vi "place_cheese_in_maze.vi"(1 "Array in":T1[][](array[typedef])) -> (0 "Array out":T1[][](array[typedef]))   [LabVIEW 2016]
doc: "Searches for the last open row of last column in the maze the places the cheese in.\n\nMuhannad Alghamdi\nCSUSB Physics 350"
uses:
  typedefs/cell_typedef.ctl
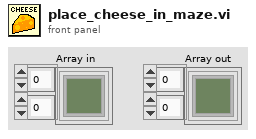
[diagram p1: front panel]
types:
  T1 = typedef "cell_typedef.ctl" = cluster{"open":bool, "runner":u16}
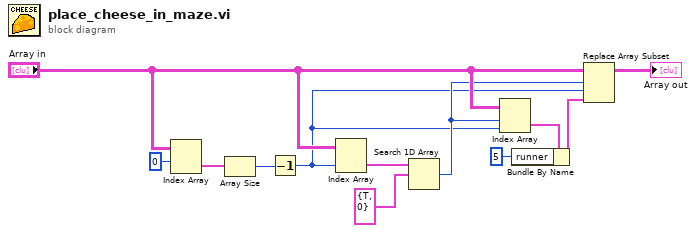
[diagram p0: block diagram]
diagram:
  n1 = Index Array(array="Array in", index (row)=0) -> (element=w6:T1[])  [unwired: 1 in]
  n2 = Array Size(array=w6) -> (size(s)=w7:i32)
  n3 = Decrement(x=w7) -> (x-1=w9:i32)
  n4 = Index Array(array="Array in", index (col)=w9) -> (element=w8:T1[])  [unwired: 1 in]
  n5 = Search 1D Array(1D array=w8, element=T1 {"open"=TRUE, "runner"=0}) -> (index of element=w10:i32)  [unwired: 1 in]
  n6 = Index Array(array="Array in", index (row)=w10, index (col)=w9) -> (element=w2:T1)
  n7 = Bundle By Name(cluster=w2, "runner"=u16 5) -> (w4:T1)
  n8 = Replace Array Subset(array="Array in", new element=w4, index (row)=w10, index (col)=w9) -> (→"Array out":T1[][])
